vi "Update FP Ctrls by mode.vi"(8 "error in (no error)":errorcluster, 9 "Mode":string, 10 "encoder to set ref":refnum<vi>, 11 "motor_parameters ref":refnum<vi>) -> (0 "error out":errorcluster)   [LabVIEW 2016, in "Hardware.lvlib" / "Motor.lvlib" / "Motor Configuration.lvclass"]
uses:
  <userlib>/Common Components/Hardware/Motor/Motor Config/Motor Configuration.lvclass
  <userlib>/Common Components/Hardware/Motor/Motor/Motor_Parameters.ctl
  <userlib>/Common Components/Hardware/Motor/Motor/Motor.lvclass
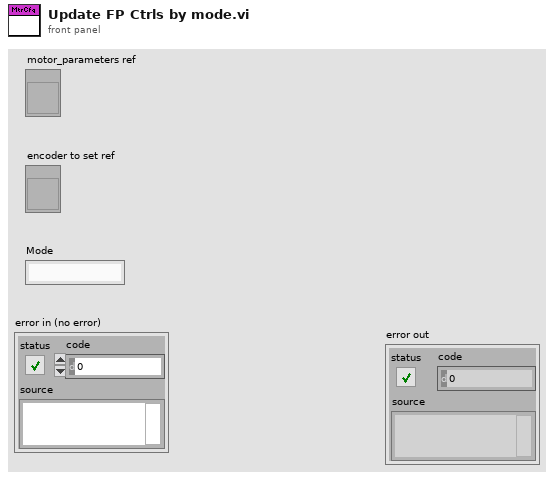
[diagram p1: front panel]
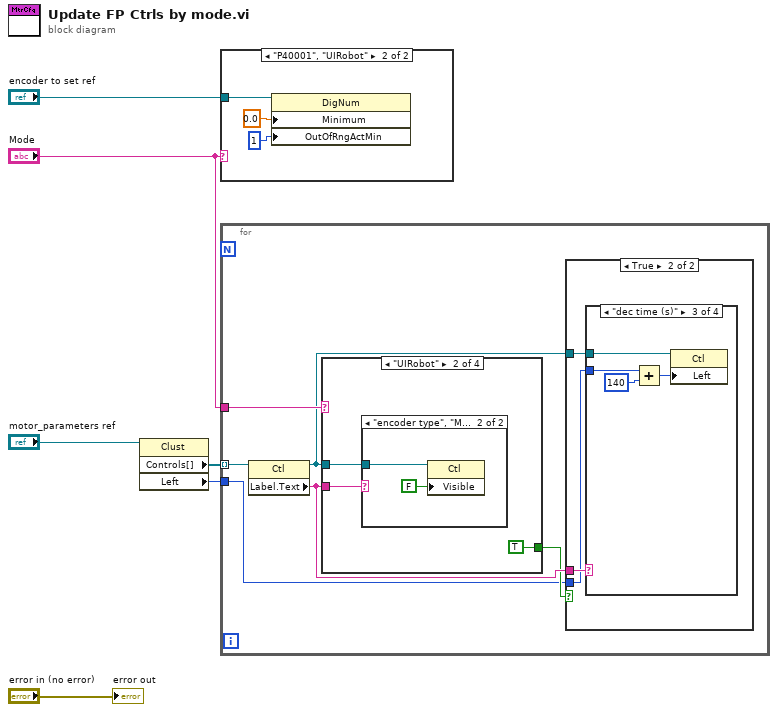
[diagram p0: block diagram]
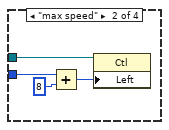
[diagram p4: hidden frame]
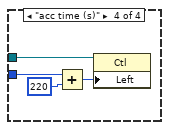
[diagram p5: hidden frame]
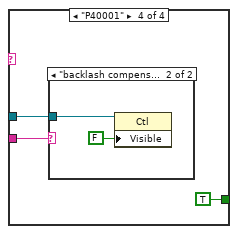
[diagram p9: hidden frame]
diagram:
  n1 = property class="Clust"(reference="motor_parameters ref") -> ("Controls[]"=w4:refnum<vi>[], "Left"=w1:i32)  [unwired: 1 in, 2 out]
  n2 = case shown="\"P40001\", \"UIRobot\"" "Mode" {
    tunnel: "encoder to set ref" -> [_ w9]
    frame Default {
    }
    frame "P40001", "UIRobot" {
      n3 = property class="DigNum"(reference=w9, "Minimum"=0.0 ("Data Entry Limits:Minimum"), "OutOfRngActMin"=u8 1 ("Response to Value Outside Limits:Minimum")) -> ()  [unwired: 1 in, 2 out]
    }
  }
  n4 = for {
    tunnel: w4 -> [w15] mode=indexing
    tunnel: "Mode" -> [w14]
    tunnel: w1 -> [w10]
    n5 = property class="Ctl"(reference=w15) -> (reference out=w12:refnum<vi>, "Label.Text"=w13:string)  [unwired: 1 in, 1 out]
    n6 = case shown="\"UIRobot\"" w14 {
      tunnel: w13 -> [_ w32 _ w38]
      tunnel: w12 -> [_ w33 _ w37]
      tunnel: [_ TRUE _ TRUE] -> w11
      frame Default {
      }
      frame "UIRobot" {
        n7 = case shown="\"encoder type\", \"Max No. of pull-ins\", \"min speed\"" w32 {
          tunnel: w33 -> [_ w35]
          frame Default {
          }
          frame "encoder type", "Max No. of pull-ins", "min speed" {
            n8 = property class="Ctl"(reference=w35, "Visible"=FALSE) -> ()  [unwired: 1 in, 2 out]
          }
        }
      }
      frame "SMC60x" {
      }
      frame "P40001" {
        n9 = case shown="\"backlash compensation\", \"backlash option\", \"encoder type\", \"Limit+\", \"Limit+ Logic\", \"Limit+ Mode\", \"Limit+ Sensor ID\", \"Limit-\", \"Limit- Logic\", \"Limit- Mode\", \"Limit- Sensor ID\", \"Max No. of pull-ins\", \"min speed\", \"soft limit max\", \"soft limit min\", \"soft offset\"" w38 {
          tunnel: w37 -> [_ w40]
          frame Default {
          }
          frame "backlash compensation", "backlash option", "encoder type", "Limit+", "Limit+ Logic", "Limit+ Mode", "Limit+ Sensor ID", "Limit-", "Limit- Logic", "Limit- Mode", "Limit- Sensor ID", "Max No. of pull-ins", "min speed", "soft limit max", "soft limit min", "soft offset" {
            n10 = property class="Ctl"(reference=w40, "Visible"=FALSE) -> ()  [unwired: 1 in, 2 out]
          }
        }
      }
    }
    n11 = case shown="True" w11 {
      tunnel: w13 -> [_ w18]
      tunnel: w12 -> [_ w17]
      tunnel: w10 -> [_ w16]
      frame False {
      }
      frame True {
        n12 = case shown="\"dec time (s)\"" w18 {
          tunnel: w17 -> [_ w22 w26 w29]
          tunnel: w16 -> [_ w19 w23 w27]
          frame Default {
          }
          frame "max speed" {
            n13 = Add(x=w19, y=8 ("Position:Left")) -> (x+y=w20:i32)
            n14 = property class="Ctl"(reference=w22, "Left"=w20) -> ()  [unwired: 1 in, 2 out]
          }
          frame "dec time (s)" {
            n15 = Add(x=w23, y=140 ("Position:Left")) -> (x+y=w25:i32)
            n16 = property class="Ctl"(reference=w26, "Left"=w25) -> ()  [unwired: 1 in, 2 out]
          }
          frame "acc time (s)" {
            n17 = Add(x=w27, y=220 ("Position:Left")) -> (x+y=w28:i32)
            n18 = property class="Ctl"(reference=w29, "Left"=w28) -> ()  [unwired: 1 in, 2 out]
          }
        }
      }
    }
  }
  "error out" <- "error in (no error)"
